vi "fstat.vi"(8 "error in (no error)":errorcluster, 11 "file descriptor":i32) -> (0 "error out":errorcluster, 3 "stat":T1)   [LabVIEW 2013, in "Linux RT IPC.lvlib" / "Shared Memory.lvlib" / "Shared Memory.lvclass"]
doc: "Wrapper VI for Linux function fstat()."
uses:
  Shared Memory.lvclass
  Controls/C Types/stat_64.ctl
  Controls/C Types/dev_t.ctl
  Controls/C Types/ino_t_64.ctl
  Controls/C Types/mode_t.ctl
  Controls/C Types/nlink_t_64.ctl
  Controls/C Types/uid_t.ctl
  Controls/C Types/gid_t.ctl
  Controls/C Types/off_t_64.ctl
  Controls/C Types/blksize_t_64.ctl
  Controls/C Types/blkcnt_t_64.ctl
  Controls/C Types/time_t_64.ctl
  Controls/C Types/stat_32.ctl
  Controls/C Types/ino_t_32.ctl
  Controls/C Types/nlink_t_32.ctl
  Controls/C Types/off_t_32.ctl
  Controls/C Types/blksize_t_32.ctl
  Controls/C Types/blkcnt_t_32.ctl
  Controls/C Types/time_t_32.ctl
  Controls/functions.ctl
  <vilib>/NI/NI Linux RT Errno/Linux Errno.lvlib
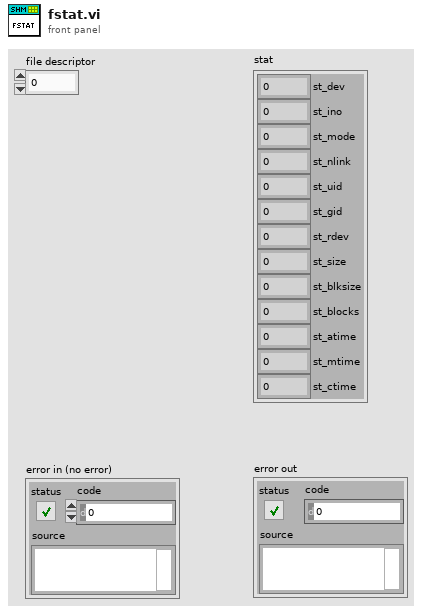
[diagram p1: front panel]
types:
  T1 = typedef "Linux RT IPC.lvlib/Shared Memory.lvlib/Shared Memory.lvclass/stat_64.ctl" = cluster{"st_dev":T2, "st_ino":T3, "st_mode":T4, "st_nlink":T5, "st_uid":T6, "st_gid":T7, "st_rdev":T2, "st_size":T8, "st_blksize":T9, "st_blocks":T10, "st_atime":T11, "st_mtime":T11, "st_ctime":T11}
  T2 = typedef "Linux RT IPC.lvlib/Shared Memory.lvlib/Shared Memory.lvclass/dev_t.ctl" = u64
  T3 = typedef "Linux RT IPC.lvlib/Shared Memory.lvlib/Shared Memory.lvclass/ino_t_64.ctl" = u64
  T4 = typedef "Linux RT IPC.lvlib/Shared Memory.lvlib/Shared Memory.lvclass/mode_t.ctl" = u32
  T5 = typedef "Linux RT IPC.lvlib/Shared Memory.lvlib/Shared Memory.lvclass/nlink_t_64.ctl" = u64
  T6 = typedef "Linux RT IPC.lvlib/Shared Memory.lvlib/Shared Memory.lvclass/uid_t.ctl" = u32
  T7 = typedef "Linux RT IPC.lvlib/Shared Memory.lvlib/Shared Memory.lvclass/gid_t.ctl" = u32
  T8 = typedef "Linux RT IPC.lvlib/Shared Memory.lvlib/Shared Memory.lvclass/off_t_64.ctl" = u64
  T9 = typedef "Linux RT IPC.lvlib/Shared Memory.lvlib/Shared Memory.lvclass/blksize_t_64.ctl" = u64
  T10 = typedef "Linux RT IPC.lvlib/Shared Memory.lvlib/Shared Memory.lvclass/blkcnt_t_64.ctl" = u64
  T11 = typedef "Linux RT IPC.lvlib/Shared Memory.lvlib/Shared Memory.lvclass/time_t_64.ctl" = u64
  T12 = typedef "Linux RT IPC.lvlib/Shared Memory.lvlib/Shared Memory.lvclass/functions.ctl" = enum16{"unspecified", "shm_open", "ftruncate", "mmap", "munmap", "close", "shm_unlink", "fstat"}
  T13 = typedef "Linux RT IPC.lvlib/Shared Memory.lvlib/Shared Memory.lvclass/stat_32.ctl" = cluster{"st_dev":T2, "st_ino":T14, "st_mode":T4, "st_nlink":T15, "st_uid":T6, "st_gid":T7, "st_rdev":T2, "st_size":T16, "st_blksize":T17, "st_blocks":T18, "st_atime":T19, "st_mtime":T19, "st_ctime":T19}
  T14 = typedef "Linux RT IPC.lvlib/Shared Memory.lvlib/Shared Memory.lvclass/ino_t_32.ctl" = u32
  T15 = typedef "Linux RT IPC.lvlib/Shared Memory.lvlib/Shared Memory.lvclass/nlink_t_32.ctl" = u32
  T16 = typedef "Linux RT IPC.lvlib/Shared Memory.lvlib/Shared Memory.lvclass/off_t_32.ctl" = u32
  T17 = typedef "Linux RT IPC.lvlib/Shared Memory.lvlib/Shared Memory.lvclass/blksize_t_32.ctl" = u32
  T18 = typedef "Linux RT IPC.lvlib/Shared Memory.lvlib/Shared Memory.lvclass/blkcnt_t_32.ctl" = u32
  T19 = typedef "Linux RT IPC.lvlib/Shared Memory.lvlib/Shared Memory.lvclass/time_t_32.ctl" = u32
  T20 = typedef "Linux Errno.lvlib/errno.ctl" = enum16{"NO ERROR", "EPERM", "ENOENT", "ESRCH", "EINTR", "EIO", "ENXIO", "E2BIG", "ENOEXEC", "EBADF", "ECHILD", "EAGAIN", "ENOMEM", "EACCES", "EFAULT", "ENOTBLK", "EBUSY", "EEXIST", "EXDEV", "ENODEV", "ENOTDIR", "EISDIR", "EINVAL", "ENFILE", "EMFILE", "ENOTTY", "ETXTBSY", "EFBIG", "ENOSPC", "ESPIPE", "EROFS", "EMLINK", "EPIPE", "EDOM", "ERANGE", "EDADLK", "ENAMETOOLONG", "ENOLCK", "ENOSYS", "ENOTEMPTY", "ELOOP", "EWOULDBLOCK", "ENOMSG", "EIDRM", "ECHRNG", "EL2NSYNC", "EL3HLT", "EL3RST", "ELNRNG", "EUNATCH", "ENOCSI", "EL2HLT", "EBADE", "EBADR", "EXFULL", "ENOANO", "EBADRQC", "EBADSLT", "EDEADLOCK", "EBFONT", "ENOSTR", "ENODATA", "ETIME", "ENOSR", "ENONET", "ENOPKG", "EREMOTE", "ENOLINK", "EADV", "ESRMNT", "ECOMM", "EPROTO", "EMULTIHOP", "EDOTDOT", "EBADMSG", "EOVERFLOW", "ENOTUNIQ", "EBADFD", "EREMCHG", "ELIBACC", "ELIBBAD", "ELIBSCN", "ELIBMAX", "ELIBEXEC", "ELISEQ", "ERESTART", "ESTRPIPE", "EUSERS", "ENOTSOCK", "EDESTADDRREQ", "EMSGSIZE", "EPROTOTYPE", "ENOPROTOOPT", "EPROTONOSUPPORT", "ESOCKTNOSUPPORT", "EOPNOTSUPP", "EPFNOSUPPORT", "EAFNOSUPPORT", "EADDRINUSE", "EADDRNOTAVAIL", "ENETDOWN", "ENETUNREACH", "ENETRESET", "ECONNABORTED", "ECONNRESET", "ENOBUFS", "EISCONN", "ENOTCONN", "ESHUTDOWN", "ETOOMANYREFS", "ETIMEDOUT", "ECONNREFUSED", "EHOSTDOWN", "EHOSTUNREACH", "EALREADY", "EINPROGRESS", "ESTALE", "EUCLEAN", "ENOTNAM", "ENAVAIL", "EISNAM", "EREMOTEIO", "EDQUOT", "ENOMEDIUM", "EMEDIUMTYPE", "ECANCELED", "ENOKEY", "EKEYEXPIRED", "EKEYREVOKED", "EKEYREJECTED", "EOWNERDEAD", "ENOTRECOVERABLE", "ERFKILL", "EHWPOISON", "UNDEFINED"}
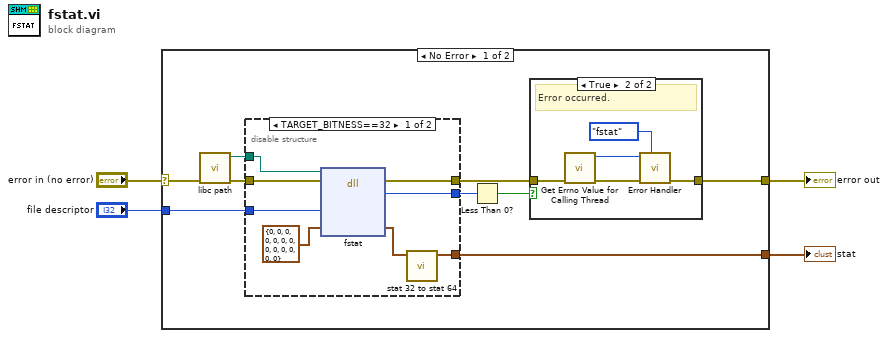
[diagram p0: block diagram]
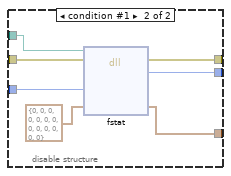
[diagram p3: hidden frame]
diagram:
  n1 = case shown="No Error" "error in (no error)" {
    selector: "error in (no error)" -> [w13 w35]
    tunnel: "file descriptor" -> [w12 _]
    tunnel: [w6 w35] -> w3
    tunnel: [w11 _] -> w1
    frame No Error {
      n2 = call "libc path.vi"("error in (no error)"=w13) -> ("error out"=w10:errorcluster, "path to libc"=w9:path)  [unwired: 9 in]
      n3 = disable-structure shown="TARGET_BITNESS==32" {
        disable-tunnel: w10 -> [w27 w34]
        disable-tunnel: w12 -> [w26 w33]
        disable-tunnel: w9 -> [w20 w32]
        disable-tunnel: [w23 w30] -> w11
        disable-tunnel: [w22 w28] -> w7
        disable-tunnel: [w21 w29] -> w8
        frame condition #0 (active) {
          n4 = dll-call lib="?" fn="fstat"(path in=w20, error in=w27, "fd"=w26, "stat"=T13 {"st_dev"=0, "st_ino"=0, "st_mode"=0, "st_nlink"=0, "st_uid"=0, "st_gid"=0, "st_rdev"=0, "st_size"=0, "st_blksize"=0, "st_blocks"=0, "st_atime"=0, "st_mtime"=0, "st_ctime"=0}) -> (error out=w22:errorcluster, "status"=w21:i32, "stat"=w24:T13)  [unwired: 2 in, 1 out]
          n5 = call "stat 32 to stat 64.vi"("stat 32"=w24) -> ("stat 64"=w23:T1)  [unwired: 10 in]
        }
        frame condition #1 {
          n6 = dll-call lib="?" fn="fstat"(path in=w32, error in=w34, "fd"=w33, "stat"=T1 {"st_dev"=0, "st_ino"=0, "st_mode"=0, "st_nlink"=0, "st_uid"=0, "st_gid"=0, "st_rdev"=0, "st_size"=0, "st_blksize"=0, "st_blocks"=0, "st_atime"=0, "st_mtime"=0, "st_ctime"=0} ("stat 2")) -> (error out=w28:errorcluster, "status"=w29:i32, "stat"=w30:T1)  [unwired: 2 in, 1 out]
        }
      }
      n7 = Less Than 0?(x=w8) -> (x < 0?=w5:bool)
      n8 = case shown="True" w5 {
        tunnel: w7 -> [w14 w19]
        tunnel: [w14 w16] -> w6
        frame False {
          # "No error."
        }
        frame True {
          # "Error occurred."
          n9 = call <vilib>:"Get Errno Value for Calling Thread.vi"("error in (no error)"=w19) -> ("error out"=w17:errorcluster, "errno"=w15:T20)  [unwired: 9 in]
          n10 = call "Error Handler.vi"("function"=functions."fstat", "error in (no error)"=w17, "errno"=w15) -> ("error out"=w16:errorcluster)  [unwired: 8 in]
        }
      }
    }
    frame Error {
    }
  }
  "error out" <- w3
  "stat" <- w1
